vi "stop.vi"(8 "error in (no error)":errorcluster, 11 "FlukeDMM in":refnum<class "FlukeDMM.lvclass">) -> (0 "error out":errorcluster, 3 "FlukeDMM out":refnum<class "FlukeDMM.lvclass">)   [LabVIEW 2013, in "FlukeDMM.lvlib" / "FlukeDMM.lvclass"]
uses:
  <userlib>/Common/Devices/FlukeDMM/FlukeDMM/FlukeDMM.lvclass
  <userlib>/Common/Devices/FlukeDMM/FlukeDMM/FlukeDMM.lvclass/FlukeDMM.ctl
  <userlib>/Common/SerialProtocols/SerialCommunicator/SerialCommunicator.lvclass
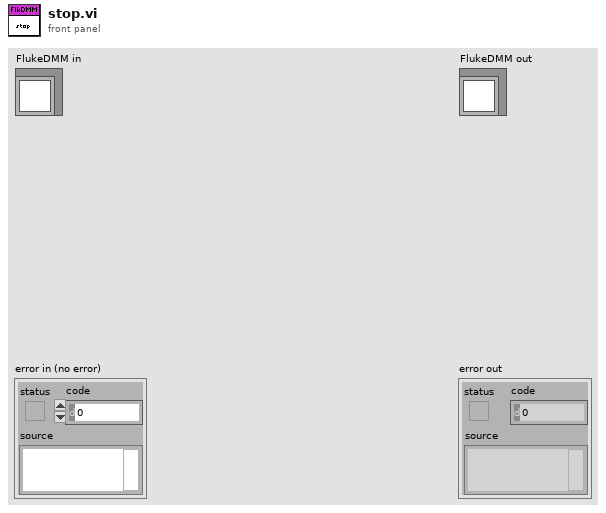
[diagram p1: front panel]
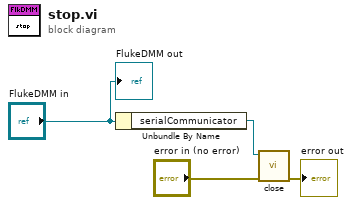
[diagram p0: block diagram]
diagram:
  n1 = Unbundle By Name("FlukeDMM in") -> ("serialCommunicator"=w4:refnum<class "SerialCommunicator.lvclass">)
  n2 = call-dynamic "close.vi"("error in (no error)"="error in (no error)", "SerialCommunicator in"=w4) -> ("error out"=→"error out":errorcluster)  [unwired: 8 in, 1 out]
  "FlukeDMM out" <- "FlukeDMM in"
